vi "TestUmgebung_aktivieren.vi"(11 "TestUmgebung aktiv/inaktiv":bool) -> (0 "Fehler (Ausgang)":errorcluster)   [LabVIEW 2020]
uses:
  Allgemein/allgemeine Sub-VIs.lvlib
  ConditionalDeactivation/ConditionalDeactivation.lvlib
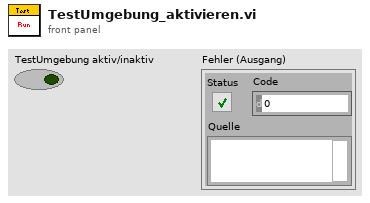
[diagram p1: front panel]
types:
  T1 = cluster{"Keys aus Projekt":string[], "Values aus Projekt":string[]}
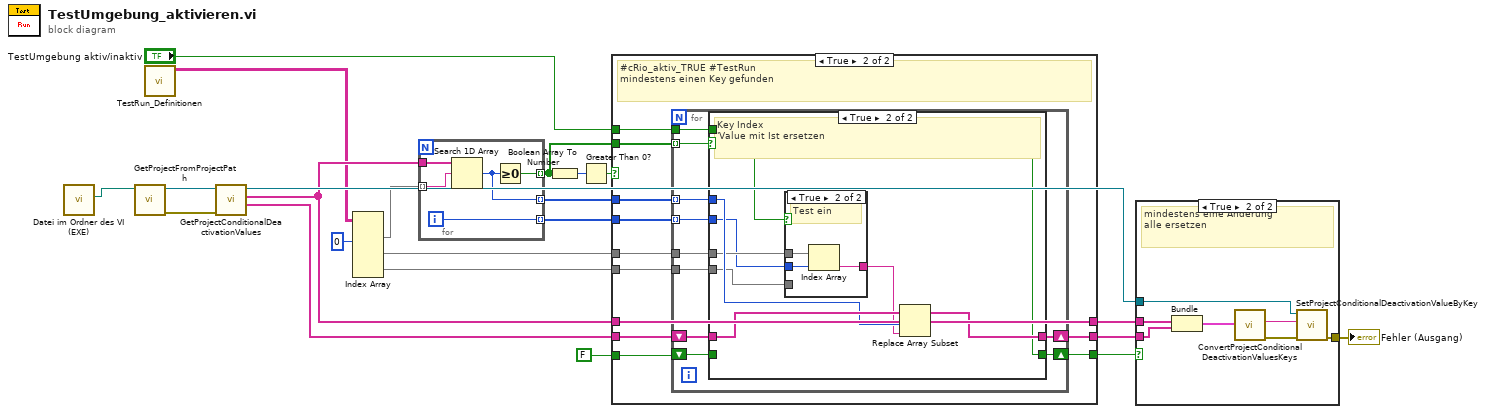
[diagram p0: block diagram]
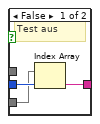
[diagram p5: hidden frame]
diagram:
  n1 = call "Datei im Ordner des VI (EXE).vi"() -> ("Ordner des Haupt-VIs"=w20:path)  [unwired: 9 in, 2 out]
  n2 = call "GetProjectFromProjectPath.vi"("ProjectPfad"=w20) -> ("Fehler (Ausgang)"=w21:errorcluster, "Projekt Referenz"=w22:refnum<vi>)  [unwired: 9 in]
  n3 = call "TestRun_Definitionen.vi"() -> ("Settings_Key_Ist_Soll"=w16:string[][])  [unwired: 11 in]
  n4 = call "GetProjectConditionalDeactivationValues.vi"("Fehler (Eingang, kein Fehler)"=w21, "Projekt Referenz"=w22) -> ("Values aus Projekt"=w17:string[], "Keys aus Projekt"=w18:string[], "Projekt Referenz"=w19:refnum<vi>)  [unwired: 5 in, 2 out]
  n5 = Index Array(array=w16, index (col) #1=0 ("Deaktivierter Index (Spalte)")) -> (element #1=w15:string[], element #2=w9:string[], element #3=w8:string[])  [unwired: 5 in]
  n6 = for {
    tunnel: w15 -> [w26] mode=indexing
    tunnel: w18 -> [w27]
    tunnel: [w25] -> w11 mode=indexing
    tunnel: [w24] -> w12 mode=indexing
    tunnel: [w23] -> w7 mode=indexing
    i -> [w23]
    n7 = Search 1D Array(1D array=w27, element=w26) -> (index of element=w24:i32)  [unwired: 1 in]
    n8 = Greater Or Equal To 0?(x=w24) -> (x >= 0?=w25:bool)
  }
  n9 = Boolean Array To Number(Boolean array=w11) -> (number=w14:u32)
  n10 = Greater Than 0?(x=w14) -> (x > 0?=w13:bool)
  n11 = case shown="True" w13 {
    tunnel: w12 -> [_ w40]
    tunnel: w11 -> [_ w41]
    tunnel: w18 -> [w29 w34]
    tunnel: w17 -> [w30 w39]
    tunnel: w9 -> [_ w37]
    tunnel: w8 -> [_ w36]
    tunnel: w7 -> [_ w38]
    tunnel: [w30 w35] -> w3
    tunnel: [w29 w34] -> w4
    tunnel: [w28 w33] -> w5
    tunnel: FALSE -> [w28 w32]
    tunnel: "TestUmgebung aktiv/inaktiv" -> [_ w31]
    frame False {
    }
    frame True {
      # "#cRio_aktiv_TRUE #TestRun\nmindestens einen Key gefunden"
      n12 = for {
        tunnel: w41 -> [w51] mode=indexing
        tunnel: w40 -> [w49] mode=indexing
        tunnel: w38 -> [w48] mode=indexing
        tunnel: w37 -> [w47]
        tunnel: w36 -> [w46]
        shift-right: [w45] -> w35
        shift-left: w39 -> [w50]
        shift-right: [w44] -> w33
        shift-left: w32 -> [w43]
        tunnel: w31 -> [w42]
        n13 = case shown="True" w51 {
          selector: w51 -> [_ w57]
          tunnel: w50 -> [w53 w62]
          tunnel: w49 -> [_ w61]
          tunnel: w48 -> [_ w59]
          tunnel: w47 -> [_ w60]
          tunnel: w46 -> [_ w55]
          tunnel: [w53 w58] -> w45
          tunnel: [w52 w57] -> w44
          tunnel: w43 -> [w52 _]
          tunnel: w42 -> [_ w54]
          frame False {
          }
          frame True {
            # "Key Index\n'Value mit Ist ersetzen"
            n14 = case shown="True" w54 {
              tunnel: w60 -> [_ w68]
              tunnel: w59 -> [w65 w67]
              tunnel: [w63 w66] -> w56
              tunnel: w55 -> [w64 _]
              frame False {
                # "Test aus"
                n15 = Index Array(array=w64, index=w65) -> (element=w63:string)
              }
              frame True {
                # "Test ein"
                n16 = Index Array(array=w68, index=w67) -> (element=w66:string)
              }
            }
            n17 = Replace Array Subset(array=w62, new element=w56, index=w61) -> (w58:string[])
          }
        }
      }
    }
  }
  n18 = case shown="True" w5 {
    tunnel: w4 -> [_ w72]
    tunnel: w3 -> [_ w71]
    tunnel: [_ w70] -> w1
    tunnel: w19 -> [_ w69]
    frame False {
    }
    frame True {
      # "mindestens eine Änderung\nalle ersetzen"
      n19 = Bundle("Keys aus Projekt"=w72, "Values aus Projekt"=w71) -> (w73:T1)  [unwired: 1 in]
      n20 = call "ConvertProjectConditionalDeactivationValuesKeys.vi"("CondDeact"=w73) -> ("Fehler (Ausgang)"=w74:errorcluster, "Tabellen-String"=w75:string)  [unwired: 9 in]
      n21 = call "SetProjectConditionalDeactivationValueByKey.vi"("Fehler (Eingang, kein Fehler)"=w74, "Tabellen-String"=w75, "Projekt Referenz"=w69) -> ("Fehler (Ausgang)"=w70:errorcluster)  [unwired: 7 in, 1 out]
    }
  }
  "Fehler (Ausgang)" <- w1
